vi "Simple Edge Detection.vi"(0 "In":bool) -> (1 "Rising Edge":bool, 2 "Falling Edge":bool)   [LabVIEW 2025]
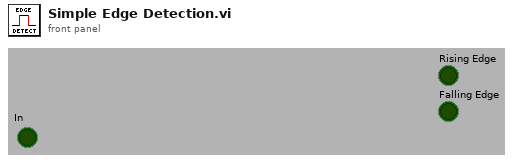
[diagram p1: front panel]
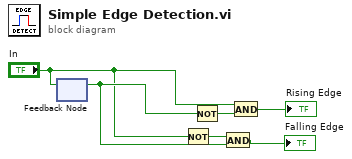
[diagram p0: block diagram]
diagram:
  n1 = feedback-in #1("In") -> ()
  n2 = feedback #1() -> (w4:bool)  [unwired: 1 in]
  n3 = Not(x="In") -> (.not. x?=w6:bool)
  n4 = Not(x=w4) -> (.not. x?=w5:bool)
  n5 = And(x=w6, y=w4) -> (x .and. y?=→"Falling Edge":bool)
  n6 = And(x="In", y=w5) -> (x .and. y?=→"Rising Edge":bool)
